vi "Read Mods.vi"(8 "error in (no error)":errorcluster, 11 "Handle Click on Graph Msg in":refnum<class "Handle Click on Graph Msg.lvclass">) -> (0 "error out":errorcluster, 2 "Mods":cluster{"Double Click":bool, "Menu Key":bool}, 3 "Handle Click on Graph Msg out":refnum<class "Handle Click on Graph Msg.lvclass">)   [LabVIEW 2020, in "GarphView.lvlib" / "Handle Click on Graph Msg.lvclass"]
uses:
  Handle Click on Graph Msg.lvclass
  Handle Click on Graph Msg.lvclass/Handle Click on Graph Msg.ctl
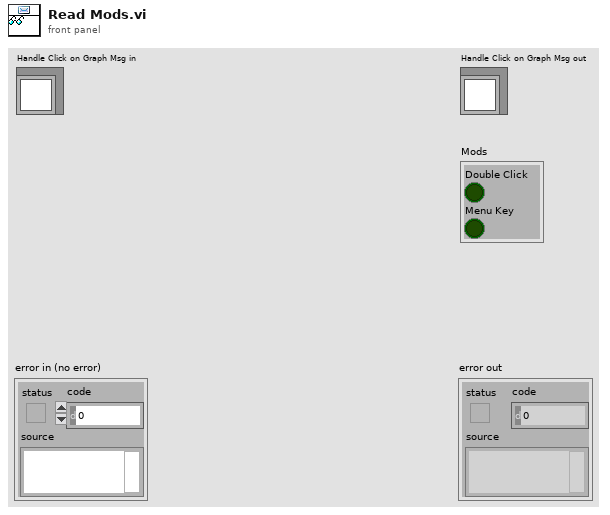
[diagram p1: front panel]
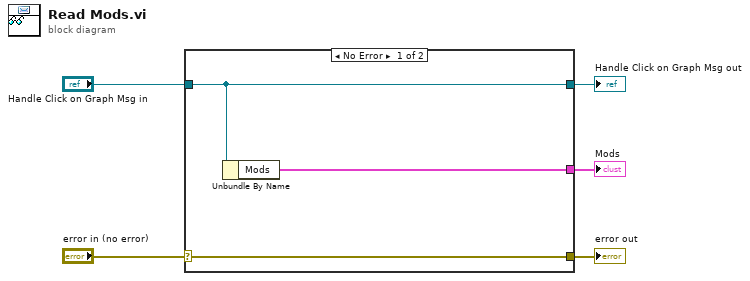
[diagram p0: block diagram]
diagram:
  n1 = case shown="No Error" "error in (no error)" {
    selector: "error in (no error)" -> [w8 w9]
    tunnel: [w8 w9] -> w4
    tunnel: [w7 w10] -> w2
    tunnel: "Handle Click on Graph Msg in" -> [w7 w10]
    tunnel: [w6 _] -> w1
    frame No Error {
      n2 = Unbundle By Name(w7) -> ("Mods"=w6:cluster{"Double Click":bool, "Menu Key":bool})
    }
    frame Error {
    }
  }
  "error out" <- w4
  "Handle Click on Graph Msg out" <- w2
  "Mods" <- w1
